vi "myRIO v1.0 Shutdown I2C.vi"(8 "error in (no error)":errorcluster, 10 "Channel":T1, 11 "myRIO Ref In":T2) -> (0 "error out":errorcluster, 3 "myRIO Ref Out":T2)   [LabVIEW 2021]
uses:
  <vilib>/myRIO/Common/Instrument Driver Framework/Utilities/typedefs/myRIO v1.0 Reference.ctl
  <vilib>/myRIO/Common/Instrument Driver Framework/Utilities/typedefs/Generic FPGA Reference.ctl
  <vilib>/myRIO/Common/Instrument Driver Framework/myRIO v1.0/I2C/typedefs/I2C Channels Enum.ctl
  <vilib>/myRIO/Common/Instrument Driver Framework/myRIO v1.0/I2C/typedefs/I2C Channels FPGA Reference.ctl
  <vilib>/rvi/errors/niLvFpgaAdjustHostInterfaceError.vi
  <vilib>/rvi/interface/nirviReadWriteControl/nirviReadWriteControl.xnode
  NiFpgaLv.dll
  <vilib>/rvi/interface/Simulation/niFpgaSimulationCallBeginRW.vi
panel:
  # "This VI turns off the specified I2C channel and zeroes out all of its registers."
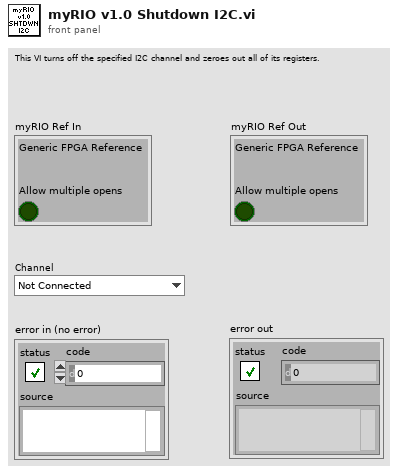
[diagram p1: front panel]
types:
  T1 = typedef "I2C Channels Enum.ctl" = enum16{"Not Connected", "A/I2C", "B/I2C", "I2C/I2C"}
  T2 = typedef "myRIO v1.0 Reference.ctl" = cluster{"Generic FPGA Reference":T3, "Allow multiple opens":bool}
  T3 = typedef "Generic FPGA Reference.ctl" = refnum<k20>
  T4 = typedef "I2C Channels FPGA Reference.ctl" = refnum<k20>
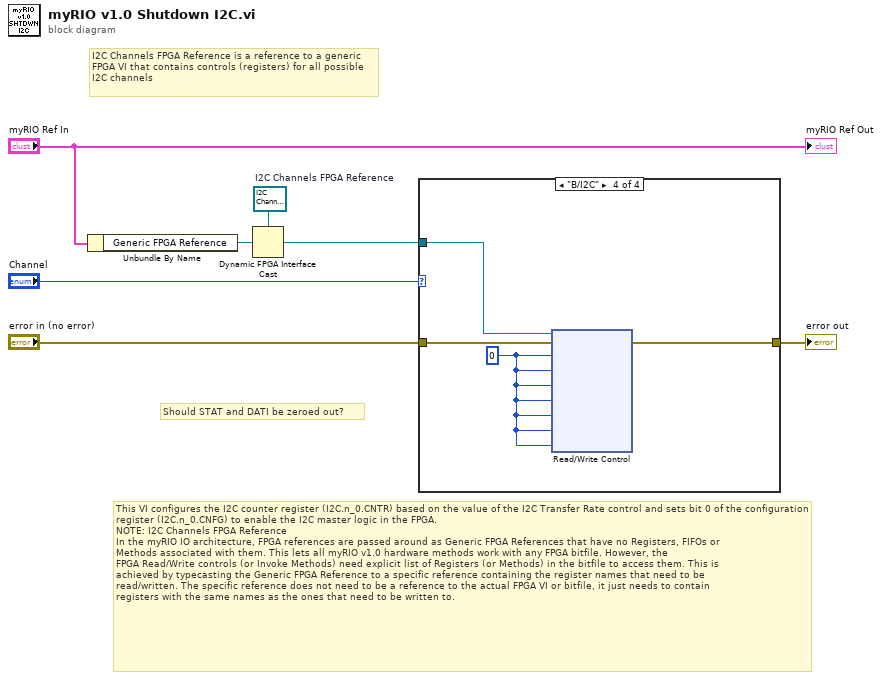
[diagram p0: block diagram]
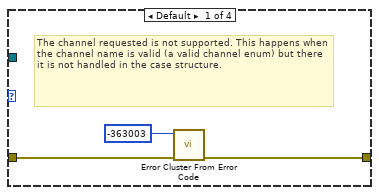
[diagram p2: hidden frame]
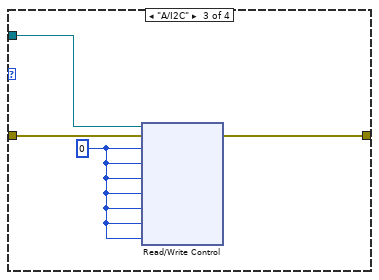
[diagram p4: hidden frame]
diagram:
  w7 = T4 refnum  # I2C Channels FPGA Reference
  # "Should STAT and DATI be zeroed out?"
  # "This VI configures the I2C counter register (I2C.n_0.CNTR) based on the value of the I2C Transfer Rate control and sets bit 0 of the configuration register (I2C.n_0.CNFG) to enable the I2C master logic in the FPGA.\nNOTE: I2C Channels FPGA Reference\nIn the myRIO IO architecture, FPGA references are passed around as Generic FPGA References that have no Registers, FIFOs or\nMethods associated with them. This lets all myRIO v1.0 hardware methods work with any FPGA bitfile. However, the \nFPGA Read/Write controls (or Invoke Methods) need explicit list of Registers (or Methods) in the bitfile to access them. This is \nachieved by typecasting the Generic FPGA Reference to a specific reference containing the register names that need to be \nread/written. The specific reference does not need to be a reference to the actual FPGA VI or bitfile, it just needs to contain \nregisters with the same names as the ones that need to be written to."
  # "I2C Channels FPGA Reference is a reference to a generic FPGA VI that contains controls (registers) for all possible I2C channels"
  n1 = Unbundle By Name("myRIO Ref In") -> ("Generic FPGA Reference"=w1:T3)
  n2 = Dynamic FPGA Interface Cast(Session In=w7, Type=w1) -> (Session Out=w6:T4)
  n3 = case shown="\"B/I2C\"" "Channel" {
    tunnel: "error in (no error)" -> [w8 w11 w14 w18]
    tunnel: [w9 w11 w13 w17] -> w3
    tunnel: w6 -> [_ _ w15 w19]
    frame Default {
      # "The channel requested is not supported. This happens when the channel name is valid (a valid channel enum) but there it is not handled in the case structure."
      n4 = call <vilib>:"Error Cluster From Error Code.vi"("error in (no error)"=w8, "error code (0)"=-363003) -> ("error out"=w9:errorcluster)  [unwired: 7 in]
    }
    frame "Not Connected" {
    }
    frame "A/I2C" {
      w12 = u8 0 ("I2C.B.CNFG")
      n5 = xnode "Read/Write Control"("FPGA VI Reference In"=w15, "error in"=w14, "I2C.A.CNFG"=w12, "I2C.A.DATO"=w12, "I2C.A.DATI"=w12, "I2C.A.ADDR"=w12, "I2C.A.CNTR"=w12, "I2C.A.CNTL"=w12, "I2C.A.STAT"=w12) -> ("error out"=w13:errorcluster)  [unwired: 1 out]
    }
    frame "B/I2C" {
      w16 = u8 0 ("I2C.B.CNFG")
      n6 = xnode "Read/Write Control"("FPGA VI Reference In"=w19, "error in"=w18, "I2C.B.CNFG"=w16, "I2C.B.DATO"=w16, "I2C.B.DATI"=w16, "I2C.B.ADDR"=w16, "I2C.B.CNTR"=w16, "I2C.B.CNTL"=w16, "I2C.B.STAT"=w16) -> ("error out"=w17:errorcluster)  [unwired: 1 out]
    }
  }
  "error out" <- w3
  "myRIO Ref Out" <- "myRIO Ref In"
